vi "Open Caller's Front Panel.vi"(0 "Open?":bool, 11 "error in (no error)":errorcluster) -> (15 "error out":errorcluster)   [LabVIEW 2020]
doc: "This vi opens the calling VI's front panel only if the calling VI has a caller itself.\n\nCoded by Douglas A. Femec, May 8, 2006.\n\nCopyright (c) 2006 MKS Instruments, Inc.\nAll rights reserved."
panel:
  # "Copyright (c) 2006 MKS Instruments, Inc.\nAll rights reserved."
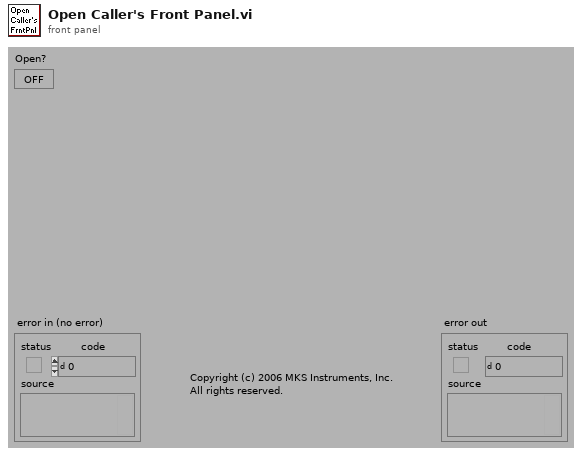
[diagram p1: front panel]
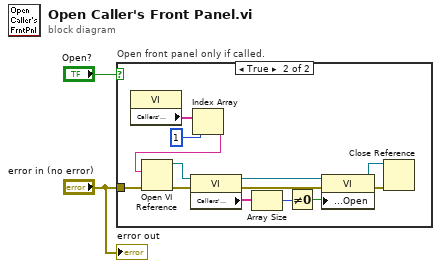
[diagram p0: block diagram]
diagram:
  n1 = case "Open front panel only if called." shown="True" "Open?" {
    tunnel: "error in (no error)" -> [_ w3]
    frame False {
    }
    frame True {
      n2 = property class="VI"() -> ("Callers' Names"=w8:string[])  [unwired: 2 in, 2 out]
      n3 = Index Array(array=w8, index=1) -> (element=w6:string)
      n4 = Open VI Reference(vi path=w6, error in (no error)=w3) -> (vi reference=w5:refnum<vi>, error out=w4:errorcluster)  [unwired: 4 in]
      n5 = property class="VI"(reference=w5, error in=w4) -> (reference out=w14:refnum<vi>, error out=w15:errorcluster, "Callers' Names"=w13:string[])
      n6 = Array Size(array=w13) -> (size(s)=w12:i32)
      n7 = Not Equal To 0?(x=w12) -> (x != 0?=w11:bool)
      n8 = property class="VI"(reference=w14, error in=w15, "Front Panel Window:Open"=w11) -> (reference out=w9:refnum<vi>, error out=w10:errorcluster)
      n9 = Close Reference(reference=w9, error in (no error)=w10) -> ()  [unwired: 1 out]
    }
  }
  "error out" <- "error in (no error)"
